vi "Main.vi"(11 "Module Admin":refnum<class "Delacor_lib_QMH_Module Admin.lvclass">) -> ()   [LabVIEW 2020, in "Settings.lvlib"]
doc: "This template is based off of the Queued Message Handler design pattern and the Queued Message Handler project template that ships with LabVIEW.\n\nThe main difference is that the queue is private to this module and communication between modules is performed via Broadcast and Request events.\n\nRequest events are wrapped in public API methods and are handled in the Event Handling Loop (EHL) of this VI. Any module can register for Broadcast events sent by this module. The EHL generates messages based on user interface actions.\n\nThe Message Handling Loop (MHL) processes messages generated by the EHL, or by other messages. The messages are string values, so new messages can be added easily to the Message Cases case structure in the MHL. Each message cluster can also provide an optional value for Message Data, which is a variant that can be converted to whatever message-specific data is required.\n_____\nBased on Delacor QMH Project Template 6.0.0.89."
uses:
  Settings.lvlib
  <vilib>/Delacor/Delacor QMH/Libraries/Module Admin_class/Delacor_lib_QMH_Module Admin.lvclass
  Aqcisition/Analog Signal Config.ctl
  Aqcisition/Digital Signal Config.ctl
  Module Data--cluster.ctl
  Stop Argument--cluster.ctl
  <vilib>/Delacor/Delacor QMH/Libraries/Message Queue_class/Delacor_lib_QMH_Message Queue.lvclass/Delacor_lib_QMH_Message Queue.ctl
  <vilib>/Delacor/Delacor QMH/Libraries/Module Admin_class/Delacor_lib_QMH_Module Admin.lvclass/Delacor_lib_QMH_Module Admin.ctl
  Save Config Argument--cluster.ctl
  Read Config Argument--cluster.ctl
  Read Config (Reply Payload)--cluster.ctl
  Save the config Argument--cluster.ctl
  Cancel config Argument--cluster.ctl
  <vilib>/Delacor/Delacor QMH/Libraries/Message Queue_class/Delacor_lib_QMH_Enqueue Message (Single).vi
  <vilib>/Delacor/Delacor QMH/Libraries/Module Admin_class/Delacor_lib_QMH_Get External Launch.vi
  <vilib>/Utility/error.llb/Error Cluster From Error Code.vi
  <vilib>/ErrorRing/Error Ring.xnode
  <vilib>/Delacor/Delacor QMH/Libraries/Message Queue_class/Delacor_lib_QMH_Message Queue.lvclass
panel:
  in  "Save Button":bool
  in  "Cancel Button":bool
  in  "Adquicision de datos":T3={"Señal Analogica"={"Canal/Canales"="", "Canal"="DAQSim1", "Canales"=[], "Frecuencia de muestreo"=1000, "Numero de muestras"=1000, "Tiempo de AQ"=0.0}, "Señal Digital"={"Puertos/Pines"="", "Puerto"="DAQSim1", "Pines"=[], "Tiempo de AQ"=0.0, "Tiempo entre AQ"=0.0}}
  out "error out":errorcluster
  out "Status":string
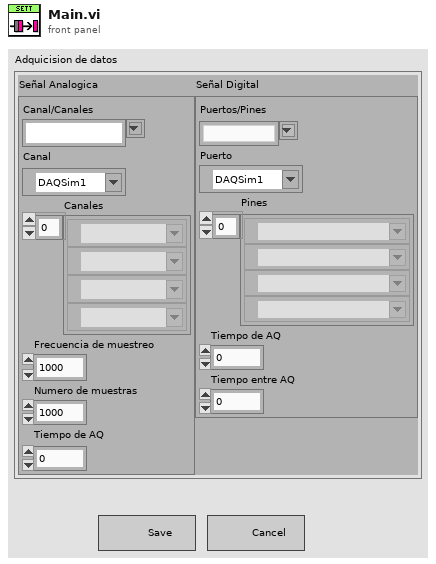
[diagram p1: front panel]
types:
  T1 = typedef "Analog Signal Config.ctl" = cluster{"Canal/Canales":string, "Canal":tag, "Canales":tag[], "Frecuencia de muestreo":i32, "Numero de muestras":i32, "Tiempo de AQ":dbl}
  T2 = typedef "Digital Signal Config.ctl" = cluster{"Puertos/Pines":string, "Puerto":tag, "Pines":tag[], "Tiempo de AQ":dbl, "Tiempo entre AQ":dbl}
  T3 = cluster{"Señal Analogica":T1, "Señal Digital":T2}
  T4 = typedef "Settings.lvlib/Request Events--cluster.ctl" = cluster{"Stop Module":refnum<user-event>, "Show Panel":refnum<user-event>, "Hide Panel":refnum<user-event>, "Get Module Execution Status":refnum<user-event>, "Show Diagram":refnum<user-event>, "Save Config":refnum<user-event>, "Read Config":refnum<user-event>, "Save the config":refnum<user-event>, "Cancel config":refnum<user-event>}
  T5 = typedef "Settings.lvlib/Module Data--cluster.ctl" = cluster{"Status":string, "Señal Analogica":T1, "Señal Digital":T2}
  T6 = enum32{"invalid lock state", "Not Locked", "Locked (No Password)", "Password-protected"}
  T7 = typedef "Settings.lvlib/Stop Argument--cluster.ctl" = cluster{"Origin":string, "Exit via Stop Module Req?":bool, "Wait for Module to stop?":bool}
  T8 = typedef "Settings.lvlib/Save Config Argument--cluster.ctl" = cluster{"Señal Analogica":T1, "Señal Digital":T2}
  T9 = typedef "Settings.lvlib/Read Config Argument--cluster.ctl" = cluster{"Wait Notifier":refnum<notifier>, "wait for reply":bool}
  T10 = typedef "Settings.lvlib/Save the config Argument--cluster.ctl" = cluster{"Save":bool}
  T11 = typedef "Settings.lvlib/Cancel config Argument--cluster.ctl" = cluster{"Cancel":bool}
  T12 = enum32{"Invalid", "Standard", "Closed", "Hidden", "Minimized", "Maximized"}
  T13 = typedef "Settings.lvlib/Read Config (Reply Payload)--cluster.ctl" = cluster{"Señal Analogica":T1, "Señal Digital":T2, "Read Config_error":errorcluster}
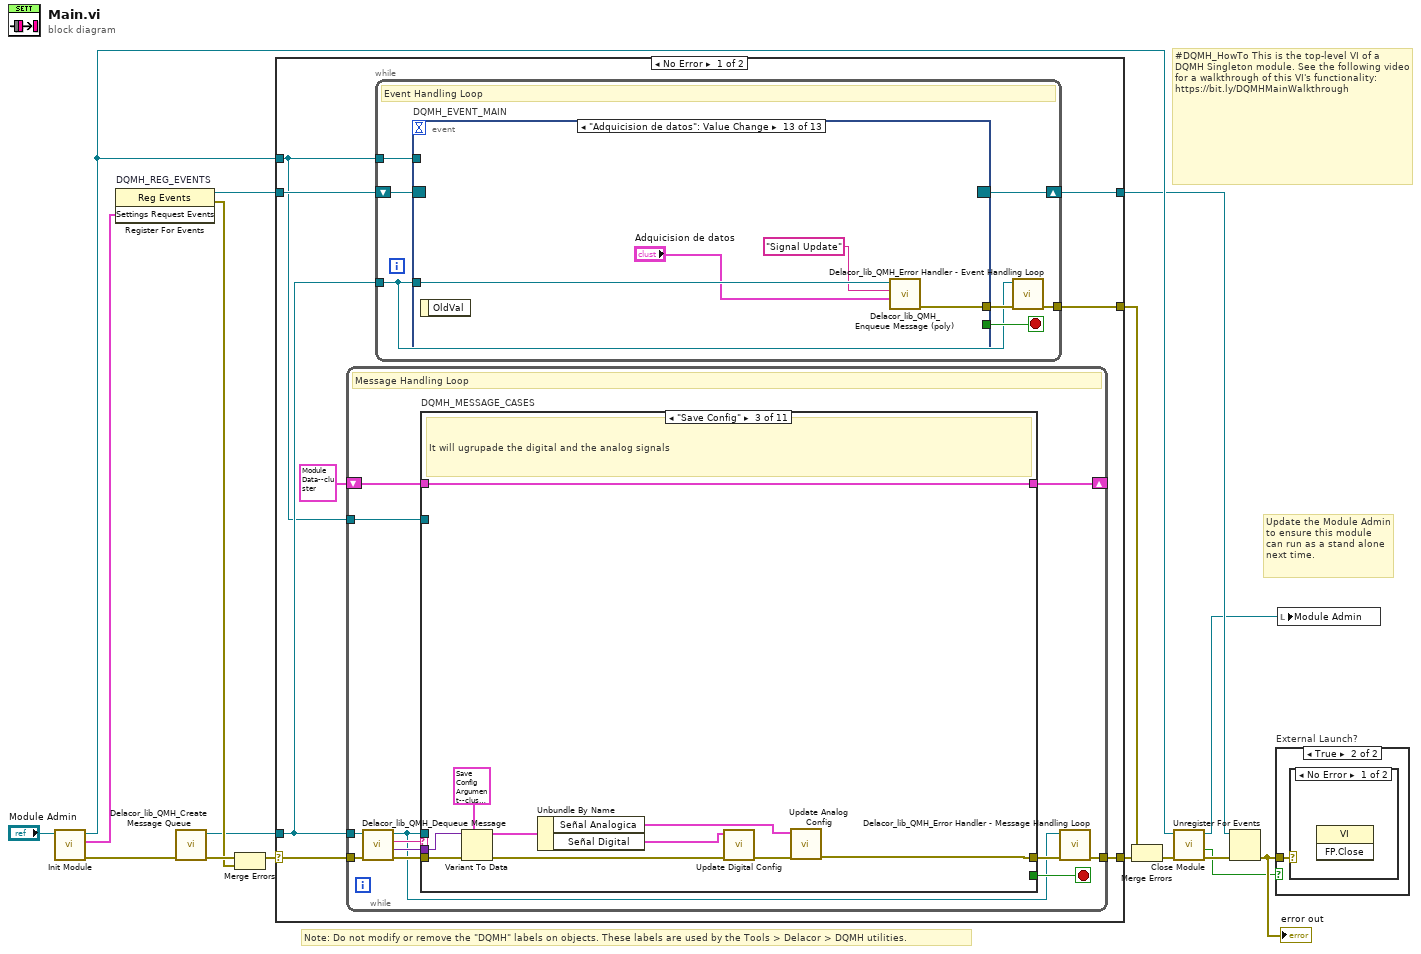
[diagram p0: block diagram]
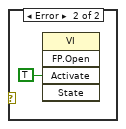
[diagram p3: hidden frame]
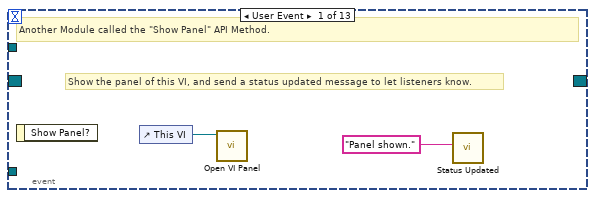
[diagram p4: hidden frame]
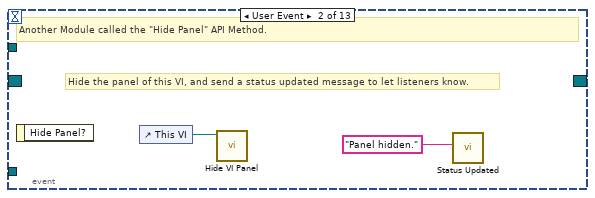
[diagram p5: hidden frame]
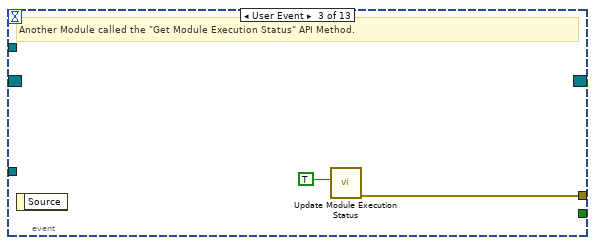
[diagram p6: hidden frame]
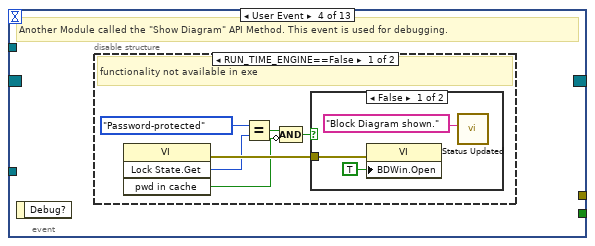
[diagram p7: hidden frame]
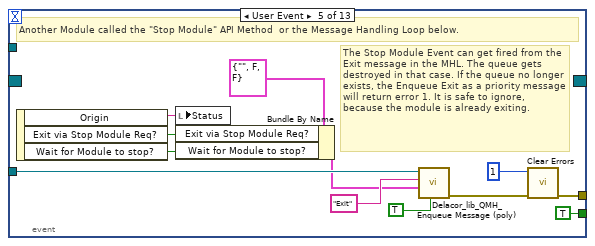
[diagram p10: hidden frame]
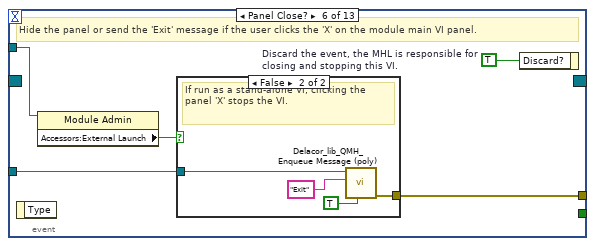
[diagram p11: hidden frame]
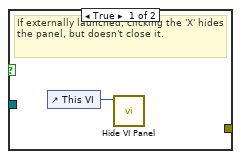
[diagram p12: hidden frame]
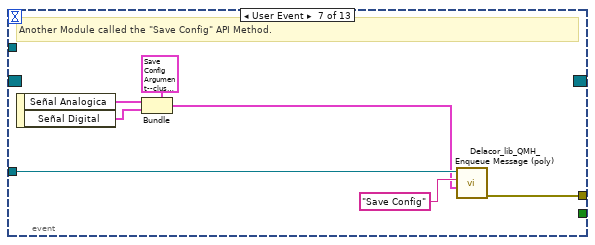
[diagram p13: hidden frame]
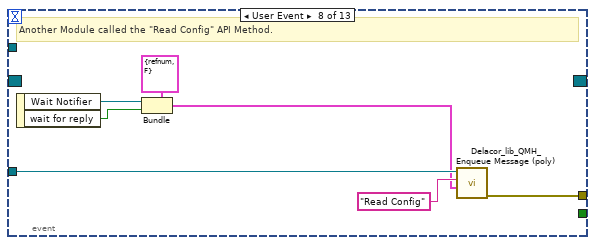
[diagram p14: hidden frame]
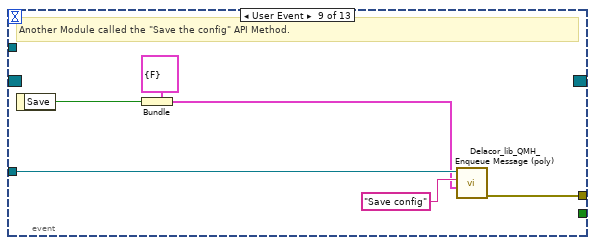
[diagram p15: hidden frame]
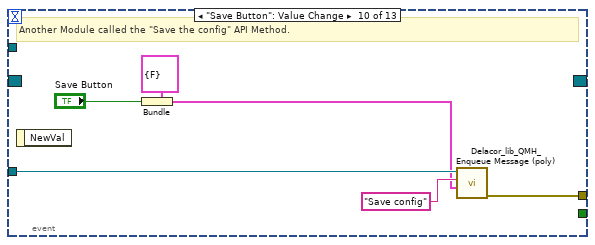
[diagram p16: hidden frame]
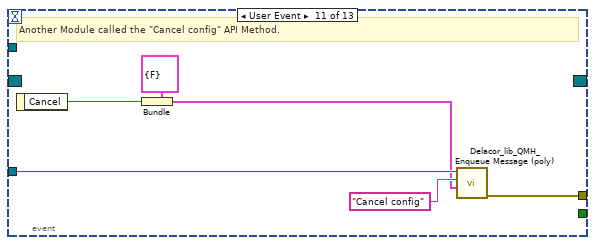
[diagram p17: hidden frame]
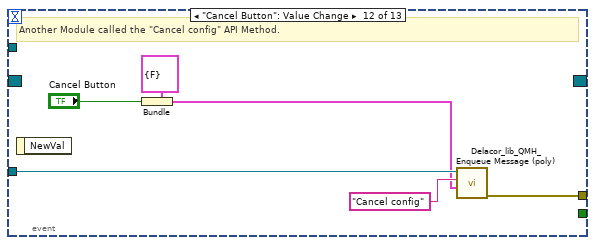
[diagram p18: hidden frame]
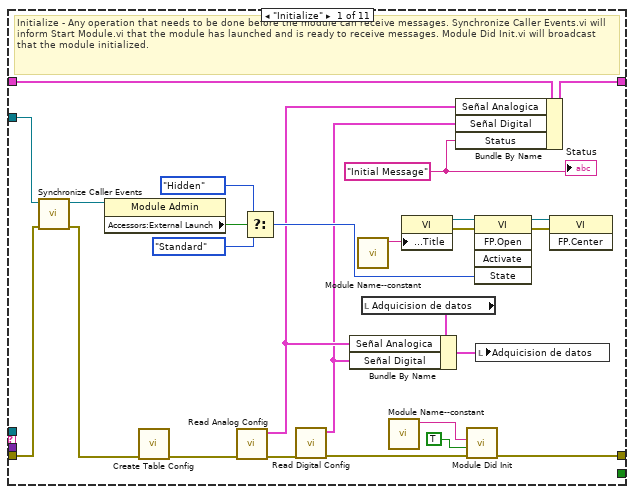
[diagram p19: hidden frame]
diagram:
  # "#DQMH_HowTo This is the top-level VI of a DQMH Singleton module. See the following video for a walkthrough of this VI's functionality: https://bit.ly/DQMHMainWalkthrough"
  # "Note: Do not modify or remove the \"DQMH\" labels on objects. These labels are used by the Tools > Delacor > DQMH utilities."
  # "Update the Module Admin to ensure this module can run as a stand alone next time."
  n1 = call "Init Module.vi"("Singleton Module Admin in"="Module Admin") -> ("error out"=w16:errorcluster, "Settings Request Events"=w5:T4, "Singleton Module Admin out"=w8:refnum<class "Delacor_lib_QMH_Module Admin.lvclass">)  [unwired: 8 in]
  n2 = register-events "DQMH_REG_EVENTS"(w5) -> (reference out=w6:refnum<event-registration>, error out=w9:errorcluster)  [unwired: 2 in]
  n3 = call <vilib>:"Delacor_lib_QMH_Create Message Queue.vi"("error in"=w16) -> ("error out"=w11:errorcluster, "Message Queue"=w4:refnum<class "Delacor_lib_QMH_Message Queue.lvclass">)  [unwired: 9 in]
  n4 = Merge Errors(w11, w9) -> (w10:errorcluster)
  n5 = case shown="No Error" w10 {
    selector: w10 -> [w23 w247]
    tunnel: [w25 w246] -> w17
    tunnel: [w22 w252] -> w7
    tunnel: w6 -> [w20 w252]
    tunnel: w4 -> [w19 w245]
    tunnel: [w24 _] -> w14
    tunnel: w8 -> [w18 w248]
    frame No Error {
      n6 = while {
        tunnel: w19 -> [w114]
        shift-right: [w118] -> _
        shift-left: T5 {"Status"="", "Señal Analogica"={"Canal/Canales"="", "Canal"="DAQSim1", "Canales"=[], "Frecuencia de muestreo"=1000, "Numero de muestras"=1000, "Tiempo de AQ"=0.0}, "Señal Digital"={"Puertos/Pines"="", "Puerto"="DAQSim1", "Pines"=[], "Tiempo de AQ"=0.0, "Tiempo entre AQ"=0.0}} ("Data Cluster") -> [w119]
        tunnel: w23 -> [w122]
        tunnel: [w120] -> w25
        tunnel: w18 -> [w112]
        stop <- w117 stop-if-true
        # "Message Handling Loop"
        n7 = call-dynamic "Delacor_lib_QMH_Dequeue Message.vi"("error in"=w122, "Message Queue in"=w114) -> ("error out"=w121:errorcluster, "Message Data"=w115:variant, "Message"=w116:string, "Message Queue out"=w113:refnum<class "Delacor_lib_QMH_Message Queue.lvclass">)  [unwired: 6 in]
        n8 = case "DQMH_MESSAGE_CASES" shown="\"Save Config\"" w116 {
          selector: w116 -> [_ _ _ _ _ _ _ _ _ _ w232]
          tunnel: w113 -> [_ _ _ _ _ _ _ _ w202 w224 _]
          tunnel: w121 -> [w147 w151 w161 w176 w185 w194 w197 w199 w209 w230 w234]
          tunnel: [w146 w151 w154 w166 w180 w192 w196 w199 w205 w227 w235] -> w123
          tunnel: w119 -> [w137 w150 w160 w175 w184 w190 w195 w198 w204 w223 w233]
          tunnel: [w136 w150 w160 w175 w184 w189 w195 w198 w204 w223 w233] -> w118
          tunnel: [_ _ _ _ _ _ _ _ _ w222 _] -> w117
          tunnel: w115 -> [_ _ w159 w173 w183 w193 _ _ w203 w221 _]
          tunnel: w112 -> [w138 _ _ _ _ _ _ _ w201 w216 _]
          frame "Initialize" {
            w132 = "Initial Message" ("Initial Message")
            # "Initialize - Any operation that needs to be done before the module can receive messages. Synchronize Caller Events.vi will inform Start Module.vi that the module has launched and is ready to receive messages. Module Did Init.vi will broadcast that the module initialized."
            n9 = call "Synchronize Caller Events.vi"("error in (no error)"=w147, "Singleton Module Admin in"=w138) -> ("error out"=w131:errorcluster, "Singleton Module Admin out"=w133:refnum<class "Delacor_lib_QMH_Module Admin.lvclass">)  [unwired: 8 in]
            n10 = property class="Module Admin"(reference=w133) -> ("Accessors:External Launch"=w142:bool)  [unwired: 1 in, 2 out]
            n11 = call "Create Table Config.vi"("error in (no error)"=w131) -> ("error out"=w130:errorcluster)  [unwired: 10 in]
            n12 = call "Read Analog Config.vi"("error in (no error)"=w130) -> ("error out"=w129:errorcluster, "Señal Analogica"=w126:T1)  [unwired: 9 in]
            n13 = Select(t=T12."Hidden" ("State"), s=w142, f=T12."Standard" ("State")) -> (s? t:f=w139:T12)
            n14 = call "Read Digital Config.vi"("error in (no error)"=w129) -> ("error out"=w128:errorcluster, "Señal Digital"=w125:T2)  [unwired: 9 in]
            n15 = call "Module Name--constant.vi"() -> ("Module Name"=w145:string)  [unwired: 11 in]
            n16 = local read "Adquicision de datos"() -> (w127:T3)
            n17 = Bundle By Name(cluster=w127, "Señal Analogica"=w126, "Señal Digital"=w125) -> (w124:T3)
            n18 = call "Module Name--constant.vi"() -> ("Module Name"=w134:string)  [unwired: 11 in]
            n19 = property class="VI"("Front Panel.Title"=w145) -> (reference out=w144:refnum<vi>, error out=w149:errorcluster)  [unwired: 2 in]
            n20 = Bundle By Name(cluster=w137, "Señal Analogica"=w126, "Señal Digital"=w125, "Status"=w132) -> (w136:T5)
            n21 = call "Module Did Init.vi"("error in (no error)"=w128, "Initialized?"=TRUE, "Origin"=w134) -> ("error out"=w146:errorcluster)  [unwired: 8 in]
            n22 = invoke class="VI" method="FP.Open"(reference=w144, error in=w149, "State"=w139) -> (reference out=w143:refnum<vi>, error out=w148:errorcluster)  [unwired: 2 in, 3 out]
            n23 = local write "Adquicision de datos"(w124) -> ()
            n24 = invoke class="VI" method="FP.Center"(reference=w143, error in=w148) -> ()  [unwired: 1 in, 3 out]
            "Status" <- w132
          }
          frame "---Module Specific---" {
            # "Separator -- The following cases handle messages specific to this Module."
          }
          frame "Save Config" {
            # "It will ugrupade the digital and the analog signals"
            n25 = Variant To Data(error in=w161, type=T8 {"Señal Analogica"={"Canal/Canales"="", "Canal"="DAQSim1", "Canales"=[], "Frecuencia de muestreo"=1000, "Numero de muestras"=1000, "Tiempo de AQ"=0.0}, "Señal Digital"={"Puertos/Pines"="", "Puerto"="DAQSim1", "Pines"=[], "Tiempo de AQ"=0.0, "Tiempo entre AQ"=0.0}} ("Save Config Argument"), Variant=w159) -> (data=w157:T8, error out=w156:errorcluster)
            n26 = Unbundle By Name(w157) -> ("Señal Analogica"=w152:T1, "Señal Digital"=w153:T2)
            n27 = call "Update Digital Config.vi"("error in (no error)"=w156, "Señal Digital"=w153) -> ("error out"=w155:errorcluster)  [unwired: 9 in]
            n28 = call "Update Analog Config.vi"("error in (no error)"=w155, "Señal Analogica"=w152) -> ("error out"=w154:errorcluster)  [unwired: 9 in]
          }
          frame "Read Config" {
            # "Read Digital and Analog info from Data Base"
            n29 = Variant To Data(error in=w176, type=T9 {"Wait Notifier"=refnum, "wait for reply"=FALSE} ("Read Config Argument"), Variant=w173) -> (data=w171:T9, error out=w174:errorcluster)
            n30 = Unbundle By Name(w171) -> ("Wait Notifier"=w170:refnum<notifier>, "wait for reply"=w169:bool)
            n31 = call "Read Analog Config.vi"() -> ("error out"=w165:errorcluster, "Señal Analogica"=w163:T1)  [unwired: 10 in]
            n32 = call "Read Digital Config.vi"("error in (no error)"=w165) -> ("error out"=w164:errorcluster, "Señal Digital"=w162:T2)  [unwired: 9 in]
            n33 = Merge Errors(w164, w174) -> (w166:errorcluster)
            n34 = Bundle By Name(cluster=T13 {"Señal Analogica"={"Canal/Canales"="", "Canal"="DAQSim1", "Canales"=[], "Frecuencia de muestreo"=1000, "Numero de muestras"=1000, "Tiempo de AQ"=0.0}, "Señal Digital"={"Puertos/Pines"="", "Puerto"="DAQSim1", "Pines"=[], "Tiempo de AQ"=0.0, "Tiempo entre AQ"=0.0}, "Read Config_error"={"status"=FALSE, "code"=0, "source"=""}} ("Read Config (Reply Payload)"), "Señal Analogica"=w163, "Señal Digital"=w162, "Read Config_error"=w164) -> (w168:T13)
            n35 = case shown="True" w169 {
              tunnel: w170 -> [_ w178]
              tunnel: w168 -> [_ w177]
              frame False {
              }
              frame True {
                n36 = Send Notification(notification=w177, notifier=w178) -> ()  [unwired: 1 in, 2 out]
              }
            }
          }
          frame "Cancel config" {
            # "Cancel every work in progress"
            n37 = Variant To Data(error in=w185, type=T11 {"Cancel"=FALSE} ("Cancel config Argument"), Variant=w183) -> (data=w181:T11, error out=w179:errorcluster)
            n38 = Unbundle By Name(w181) -> ()  [unwired: 1 out]
            n39 = call "Hide Panel.vi"("error in (no error)"=w179) -> ("error out"=w180:errorcluster)  [unwired: 10 in]
          }
          frame "Signal Update" {
            # "Cancel every work in progress"
            n40 = Variant To Data(error in=w194, type=T8 {"Señal Analogica"={"Canal/Canales"="", "Canal"="DAQSim1", "Canales"=[], "Frecuencia de muestreo"=1000, "Numero de muestras"=1000, "Tiempo de AQ"=0.0}, "Señal Digital"={"Puertos/Pines"="", "Puerto"="DAQSim1", "Pines"=[], "Tiempo de AQ"=0.0, "Tiempo entre AQ"=0.0}} ("Save Config Argument"), Variant=w193) -> (data=w191:T8, error out=w192:errorcluster)
            n41 = Unbundle By Name(w191) -> ("Señal Analogica"=w188:T1, "Señal Digital"=w187:T2)
            n42 = Bundle By Name(cluster=w190, "Señal Analogica"=w188, "Señal Digital"=w187) -> (w189:T5)
          }
          frame "---Copy This Frame---" {
            # "Duplicate this frame when creating new messages.  Change this comment in the duplicated frame to describe this message."
            n43 = Merge Errors(w197) -> (w196:errorcluster)
          }
          frame "---Exit and Error Handling---" {
            # "Separator - The following cases handle errors and exit messages."
          }
          frame "Error" {
            # "#CodeRecommended - If you ever change the name of this \"Error\" message, you'll need to update the name in the Check Loop Error.vi as well."
            # "#CodeRecommended - If the module is running in standalone mode (External Launch = FALSE), this code will pop up an error dialog and call the 'Exit' message if an error occurs. Add more fine-grained error handling here."
            # "Error - Check the error message data and respond accordingly. This message is sent by the \"Error Handler\" VIs at the end of each loop in this application."
            n44 = property class="Module Admin"(reference=w201) -> ("Accessors:External Launch"=w200:bool)  [unwired: 1 in, 2 out]
            n45 = Variant To Data(error in=w209, type=errorcluster {"status"=FALSE, "code"=0, "source"=""} ("error constant"), Variant=w203) -> (data=w210:errorcluster, error out=w207:errorcluster)
            n46 = call "Error Reported.vi"("Error"=w210) -> ()  [unwired: 10 in, 1 out]
            n47 = case shown="False" w200 {
              tunnel: [w215 _] -> w206
              tunnel: w202 -> [w213 _]
              tunnel: w210 -> [w214 _]
              frame False {
                # "If the module is running standalone, then pop up an error dialog and call the \"Exit\" message."
                n48 = call <vilib>:"Simple Error Handler.vi"("error in (no error)"=w214) -> ()  [unwired: 4 in, 5 out]
                n49 = call-poly <vilib>:"Delacor_lib_QMH_Enqueue Message (poly).vi"("Priority Message? (F)"=TRUE, "Message"="Exit", "Message Queue in"=w213) -> ("error out"=w215:errorcluster)  [unwired: 7 in, 1 out]
              }
              frame True {
                # "If the module was launched externally, calling the Error Reported broadcast VI is the only action performed by the \"Error\" message. The module's caller can then process the error appropriately."
              }
            }
            n50 = Merge Errors(w207, w206) -> (w205:errorcluster)
            n51 = local write "error out"(w205) -> ()
          }
          frame "Exit" {
            w220 = 91  # 91: not all Exit messages will have an argument
            w222 = TRUE  # Stop the VI
            # "Release the message queue reference"
            # "#CodeNeeded - Add any required cleanup code here"
            # "Exit - Exit the application."
            n52 = Variant To Data(error in=w230, type=T7 {"Origin"="", "Exit via Stop Module Req?"=FALSE, "Wait for Module to stop?"=FALSE} ("Stop Argument"), Variant=w221) -> (data=w218:T7, error out=w226:errorcluster)
            n53 = call <vilib>:"Clear Errors.vi"("error in (no error)"=w226, "specific error code to clear (0: all)"=w220) -> ("error out"=w229:errorcluster)  [unwired: 4 in, 1 out]
            n54 = control-ref of="This VI"() -> (w217:refnum<vi>)
            n55 = call-dynamic "Delacor_lib_QMH_Release Message Queue.vi"("error in"=w229, "Message Queue"=w224) -> ("error out"=w228:errorcluster)  [unwired: 9 in]
            n56 = call "Handle Exit.vi"("Stop Argument"=w218, "Admin in"=w216, "VI reference"=w217) -> ("error out"=w225:errorcluster)  [unwired: 7 in, 1 out]
            n57 = Merge Errors(w228, w225) -> (w227:errorcluster)
          }
          frame Default {
            # "'Default' case only runs if there is a message that isn't defined in any of the other cases.  Output a programming error."
            n58 = call "Module Name--constant.vi"() -> ("Module Name"=w231:string)  [unwired: 11 in]
            n59 = xnode "Error Ring"("parameter 0"=w232, "parameter 1"=w231) -> ("error out"=w236:errorcluster)
            n60 = Merge Errors(w234, w236) -> (w235:errorcluster)
          }
        }
        n61 = call-dynamic "Delacor_lib_QMH_Error Handler - Message Handling Loop.vi"("error in"=w123, "Message Queue in"=w113) -> ("dup error in"=w120:errorcluster)  [unwired: 8 in, 1 out]
      }
      n62 = while {
        tunnel: w19 -> [w26]
        shift-right: [w29] -> w22
        shift-left: w20 -> [w30]
        tunnel: [w31] -> w24
        tunnel: w18 -> [w27]
        stop <- w28 stop-if-true
        # "Event Handling Loop"
        n63 = event "DQMH_EVENT_MAIN" shown="[12] \"Adquicision de datos\": Value Change" {
          selector: w30 -> [_ _ _ _ _ _ _ _ _ _ _ _ _]
          dyn-events: [_ _ _ _ _ _ _ _ _ _ _ _ _] -> w29
          timeout: _ -> [_ _ _ _ _ _ _ _ _ _ _ _ _]
          tunnel: [_ _ _ _ TRUE ("Discard?") _ _ _ _ _ _ _ _] -> w28
          tunnel: w26 -> [_ _ _ _ w55 w62 w76 w83 w89 w95 w101 w107 w110]
          tunnel: [_ _ w38 _ w58 w64 w70 w77 w84 w91 w96 w103 w111] -> w32
          tunnel: w27 -> [_ _ _ _ _ w61 _ _ _ _ _ _ _]
          event User Event {
            # "Show the panel of this VI, and send a status updated message to let listeners know."
            # "Another Module called the \"Show Panel\" API Method."
            n64 = event-data() -> ()  [unwired: 1 in, 1 out]
            n65 = control-ref of="This VI"() -> (w34:refnum<vi>)
            n66 = call "Open VI Panel.vi"("VI"=w34) -> ()  [unwired: 10 in, 1 out]
            n67 = call "Status Updated.vi"("Status"="Panel shown." ("format string")) -> ()  [unwired: 10 in, 1 out]
          }
          event User Event {
            # "Hide the panel of this VI, and send a status updated message to let listeners know."
            # "Another Module called the \"Hide Panel\" API Method."
            n68 = event-data() -> ()  [unwired: 1 in, 1 out]
            n69 = control-ref of="This VI"() -> (w36:refnum<vi>)
            n70 = call "Hide VI Panel.vi"("VI"=w36) -> ()  [unwired: 10 in, 1 out]
            n71 = call "Status Updated.vi"("Status"="Panel hidden." ("format string")) -> ()  [unwired: 10 in, 1 out]
          }
          event User Event {
            # "Another Module called the \"Get Module Execution Status\" API Method."
            n72 = event-data() -> ()  [unwired: 1 in, 1 out]
            n73 = call "Update Module Execution Status.vi"("Running?"=TRUE) -> ("error out"=w38:errorcluster)  [unwired: 10 in]
          }
          event User Event {
            # "Another Module called the \"Show Diagram\" API Method. This event is used for debugging."
            n74 = event-data() -> ()  [unwired: 1 in, 1 out]
            n75 = disable-structure shown="RUN_TIME_ENGINE==False" {
              frame condition #0 (active) {
                # "functionality not available in exe"
                n76 = invoke class="VI" method="Lock State.Get"() -> (error out=w44:errorcluster, "Get Lock State"=w43:T6, "pwd in cache"=w40:bool)  [unwired: 4 in, 1 out]
                n77 = Equal?(x=T6."Password-protected", y=w43) -> (x = y?=w41:bool)
                n78 = Compound Arithmetic op=AND(w41, invert w40) -> (w39:bool)
                n79 = case shown="False" w39 {
                  tunnel: w44 -> [w47 _]
                  frame False {
                    n80 = property class="VI"(error in=w47, "BDWin.Open"=TRUE ("Block Diagram Window:Open")) -> ()  [unwired: 1 in, 2 out]
                    n81 = call "Status Updated.vi"("Status"="Block Diagram shown." ("format string")) -> ()  [unwired: 10 in, 1 out]
                  }
                  frame True {
                    # "Password-protected VI, and the password is not in the cache. Do not show the diagram."
                  }
                }
              }
              frame condition #1 {
              }
            }
          }
          event User Event {
            # "The Stop Module Event can get fired from the Exit message in the MHL. The queue gets destroyed in that case. If the queue no longer exists, the Enqueue Exit as a priority message will return error 1. It is safe to ignore, because the module is already exiting."
            # "Another Module called the \"Stop Module\" API Method  or the Message Handling Loop below."
            n82 = event-data() -> ("Origin"=w54:string, "Exit via Stop Module Req?"=w50:bool, "Wait for Module to stop?"=w49:bool)  [unwired: 1 in]
            n83 = local write "Status"(w54) -> ()
            n84 = Bundle By Name(cluster=T7 {"Origin"="", "Exit via Stop Module Req?"=FALSE, "Wait for Module to stop?"=FALSE} ("Stop Argument"), "Exit via Stop Module Req?"=w50, "Wait for Module to stop?"=w49) -> (w48:T7)
            n85 = call-poly <vilib>:"Delacor_lib_QMH_Enqueue Message (poly).vi"("Priority Message? (F)"=TRUE, "Message Data"=w48, "Message"="Exit", "Message Queue in"=w55) -> ("error out"=w59:errorcluster)  [unwired: 6 in, 1 out]
            n86 = call <vilib>:"Clear Errors.vi"("error in (no error)"=w59, "specific error code to clear (0: all)"=1) -> ("error out"=w58:errorcluster)  [unwired: 4 in, 1 out]
          }
          event Panel Close? {
            w63 = TRUE  # Discard the event, the MHL is responsible for closing and stopping this VI.
            # "Hide the panel or send the 'Exit' message if the user clicks the 'X' on the module main VI panel."
            n87 = event-data() -> ()  [unwired: 1 in, 1 out]
            n88 = property class="Module Admin"(reference=w61) -> ("Accessors:External Launch"=w60:bool)  [unwired: 1 in, 2 out]
            n89 = case shown="False" w60 {
              tunnel: w62 -> [_ w68]
              tunnel: [_ w69] -> w64
              frame True {
                # "If externally launched, clicking the 'X' hides the panel, but doesn't close it."
                n90 = control-ref of="This VI"() -> (w65:refnum<vi>)
                n91 = call "Hide VI Panel.vi"("VI"=w65) -> ()  [unwired: 10 in, 1 out]
              }
              frame False {
                # "If run as a stand-alone VI, clicking the panel 'X' stops the VI."
                n92 = call-poly <vilib>:"Delacor_lib_QMH_Enqueue Message (poly).vi"("Priority Message? (F)"=TRUE, "Message"="Exit", "Message Queue in"=w68) -> ("error out"=w69:errorcluster)  [unwired: 7 in, 1 out]
              }
            }
            n93 = event-data("Discard?"=w63) -> ()  [unwired: 1 in, 1 out]
          }
          event User Event {
            # "Another Module called the \"Save Config\" API Method."
            n94 = event-data() -> ("Señal Analogica"=w72:T1, "Señal Digital"=w71:T2)  [unwired: 1 in]
            n95 = Bundle(cluster=T8 {"Señal Analogica"={"Canal/Canales"="", "Canal"="DAQSim1", "Canales"=[], "Frecuencia de muestreo"=1000, "Numero de muestras"=1000, "Tiempo de AQ"=0.0}, "Señal Digital"={"Puertos/Pines"="", "Puerto"="DAQSim1", "Pines"=[], "Tiempo de AQ"=0.0, "Tiempo entre AQ"=0.0}} ("Save Config Argument"), "Señal Analogica"=w72, "Señal Digital"=w71) -> (w73:T8)
            n96 = call-poly <vilib>:"Delacor_lib_QMH_Enqueue Message (poly).vi"("Message Data"=w73, "Message"="Save Config", "Message Queue in"=w76) -> ("error out"=w70:errorcluster)  [unwired: 7 in, 1 out]
          }
          event User Event {
            # "Another Module called the \"Read Config\" API Method."
            n97 = event-data() -> ("Wait Notifier"=w79:refnum<notifier>, "wait for reply"=w78:bool)  [unwired: 1 in]
            n98 = Bundle(cluster=T9 {"Wait Notifier"=refnum, "wait for reply"=FALSE} ("Read Config Argument"), "Wait Notifier"=w79, "wait for reply"=w78) -> (w80:T9)
            n99 = call-poly <vilib>:"Delacor_lib_QMH_Enqueue Message (poly).vi"("Message Data"=w80, "Message"="Read Config", "Message Queue in"=w83) -> ("error out"=w77:errorcluster)  [unwired: 7 in, 1 out]
          }
          event User Event {
            # "Another Module called the \"Save the config\" API Method."
            n100 = event-data() -> ("Save"=w85:bool)  [unwired: 1 in]
            n101 = Bundle(cluster=T10 {"Save"=FALSE} ("Save the config Argument"), "Save"=w85) -> (w86:T10)
            n102 = call-poly <vilib>:"Delacor_lib_QMH_Enqueue Message (poly).vi"("Message Data"=w86, "Message"="Save config", "Message Queue in"=w89) -> ("error out"=w84:errorcluster)  [unwired: 7 in, 1 out]
          }
          event "Save Button": Value Change {
            # "Another Module called the \"Save the config\" API Method."
            n103 = event-data() -> ()  [unwired: 1 in, 1 out]
            n104 = Bundle(cluster=T10 {"Save"=FALSE} ("Save the config Argument"), "Save"="Save Button") -> (w92:T10)
            n105 = call-poly <vilib>:"Delacor_lib_QMH_Enqueue Message (poly).vi"("Message Data"=w92, "Message"="Save config", "Message Queue in"=w95) -> ("error out"=w91:errorcluster)  [unwired: 7 in, 1 out]
          }
          event User Event {
            # "Another Module called the \"Cancel config\" API Method."
            n106 = event-data() -> ("Cancel"=w97:bool)  [unwired: 1 in]
            n107 = Bundle(cluster=T11 {"Cancel"=FALSE} ("Cancel config Argument"), "Cancel"=w97) -> (w98:T11)
            n108 = call-poly <vilib>:"Delacor_lib_QMH_Enqueue Message (poly).vi"("Message Data"=w98, "Message"="Cancel config", "Message Queue in"=w101) -> ("error out"=w96:errorcluster)  [unwired: 7 in, 1 out]
          }
          event "Cancel Button": Value Change {
            # "Another Module called the \"Cancel config\" API Method."
            n109 = event-data() -> ()  [unwired: 1 in, 1 out]
            n110 = Bundle(cluster=T11 {"Cancel"=FALSE} ("Cancel config Argument"), "Cancel"="Cancel Button") -> (w104:T11)
            n111 = call-poly <vilib>:"Delacor_lib_QMH_Enqueue Message (poly).vi"("Message Data"=w104, "Message"="Cancel config", "Message Queue in"=w107) -> ("error out"=w103:errorcluster)  [unwired: 7 in, 1 out]
          }
          event "Adquicision de datos": Value Change {
            n112 = event-data() -> ()  [unwired: 1 in, 1 out]
            n113 = call-poly <vilib>:"Delacor_lib_QMH_Enqueue Message (poly).vi"("Message Data"="Adquicision de datos", "Message"="Signal Update", "Message Queue in"=w110) -> ("error out"=w111:errorcluster)  [unwired: 7 in, 1 out]
          }
        }
        n114 = call-dynamic "Delacor_lib_QMH_Error Handler - Event Handling Loop.vi"("error in"=w32, "Message Queue in"=w26) -> ("dup error in"=w31:errorcluster)  [unwired: 8 in, 1 out]
      }
    }
    frame Error {
      # "Synchronize Caller Events.vi will inform Start Module.vi that the module has launched and will let the code calling Start Module.vi register for broadcasts and would permit the caller receive the broadcast that an error occurred at launch time."
      n115 = call-dynamic "Delacor_lib_QMH_Release Message Queue.vi"("error in"=w247, "Message Queue"=w245) -> ("error out"=w246:errorcluster)  [unwired: 9 in]
      n116 = call "Synchronize Caller Events.vi"("Singleton Module Admin in"=w248) -> ("error out"=w253:errorcluster)  [unwired: 9 in, 1 out]
      n117 = call "Module Name--constant.vi"() -> ("Module Name"=w251:string)  [unwired: 11 in]
      n118 = Format Into String(format string="An error occurred during initialization. %s is no longer running.", w251) -> (resulting string=w249:string)  [unwired: 2 in, 1 out]
      n119 = Merge Errors(w246, w253) -> (w254:errorcluster)
      n120 = call "Error Reported.vi"("Additional Information"=w249, "Error"=w254) -> ()  [unwired: 9 in, 1 out]
    }
  }
  n121 = Merge Errors(w14, w17) -> (w13:errorcluster)
  n122 = call "Close Module.vi"("error in (no error)"=w13, "Module Admin in"=w8) -> ("error out"=w15:errorcluster, "External Launch"=w1:bool, "Module Admin out"=w2:refnum<class "Delacor_lib_QMH_Module Admin.lvclass">)  [unwired: 7 in]
  n123 = Unregister For Events(event registration refnum=w7, error in=w15) -> (error out=w12:errorcluster)
  "error out" <- w12
  n124 = case "External Launch?" shown="True" w1 {
    tunnel: w12 -> [_ w255]
    frame False {
    }
    frame True {
      n125 = case shown="No Error" w255 {
        frame No Error {
          n126 = invoke class="VI" method="FP.Close"() -> ()  [unwired: 3 in, 3 out]
        }
        frame Error {
          n127 = invoke class="VI" method="FP.Open"("Activate"=TRUE ("Activate?")) -> ()  [unwired: 4 in, 5 out]
        }
      }
    }
  }
  n128 = local write "Module Admin"(w2) -> ()
